vi "Non-Blocking Wait with Abort -- JKI SM Example.vi"() -> ()   [LabVIEW 2013]
panel:
  out "Current State":string
  out "Wait Timer Elapsed":bool
  out "Time Remaining":u32
  in  "Recipe Run Time (s)":dbl
  in  "Stop":bool
  in  "Start":bool
  in  "Exit":bool
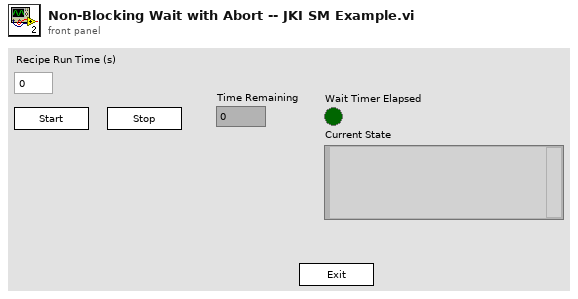
[diagram p1: front panel]
types:
  T1 = enum32{"Invalid", "Standard", "Closed", "Hidden", "Minimized", "Maximized"}
  T2 = enum32{"invalid app kind", "Development System", "Run Time System", "Student Edition", "Embedded LabVIEW", "Evaluation", "Custom"}
  T3 = cluster{"Core":cluster{"Current VI Reference":refnum<vi>, "Close Panel on Exit?":bool}, "Your Boolean data":bool, "Your string data":string}
  T4 = cluster{"Current VI Reference":refnum<vi>, "Close Panel on Exit?":bool}
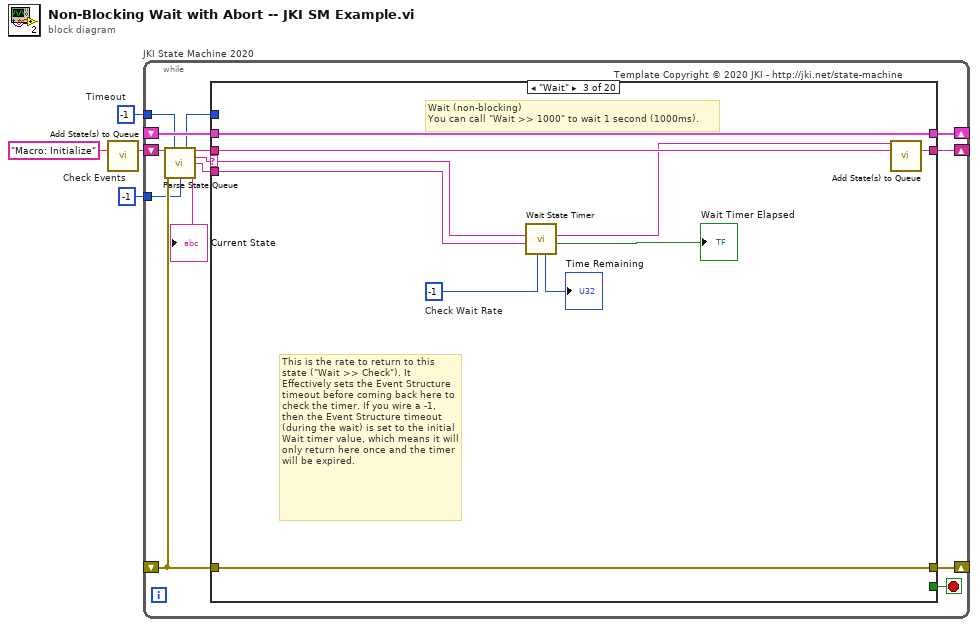
[diagram p0: block diagram]
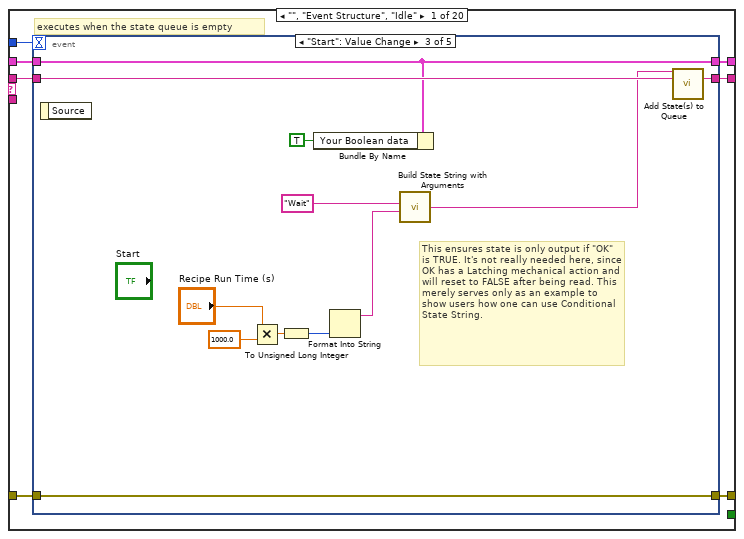
[diagram p2: hidden frame]
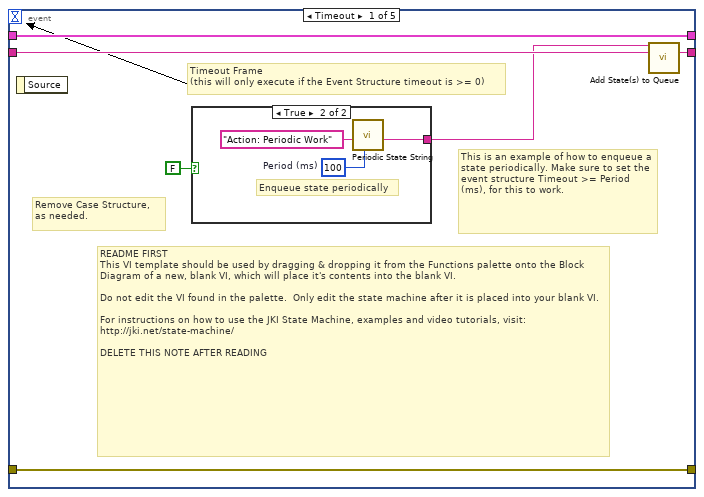
[diagram p3: hidden frame]
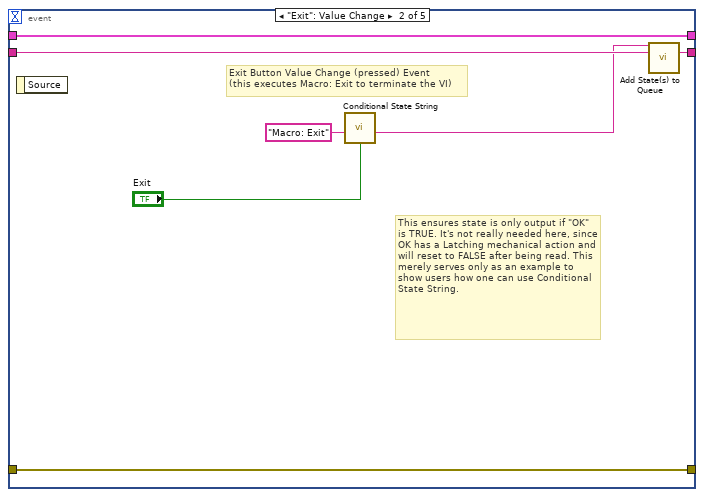
[diagram p5: hidden frame]
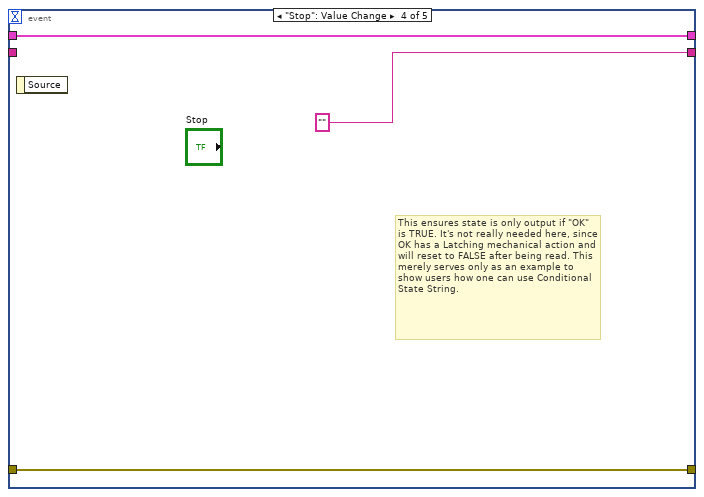
[diagram p6: hidden frame]
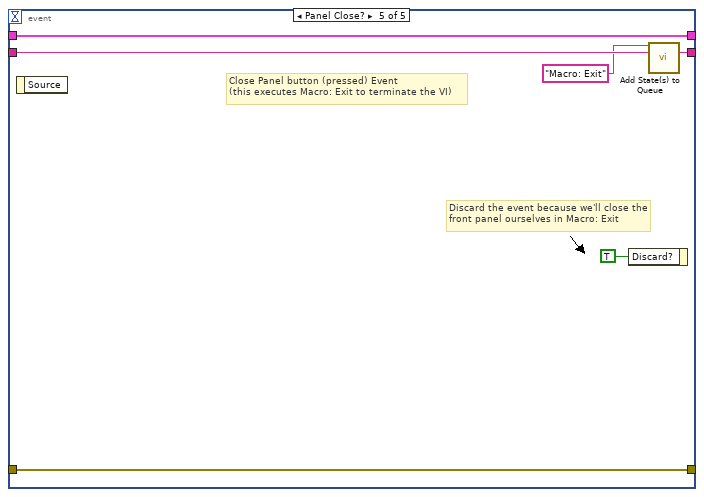
[diagram p7: hidden frame]
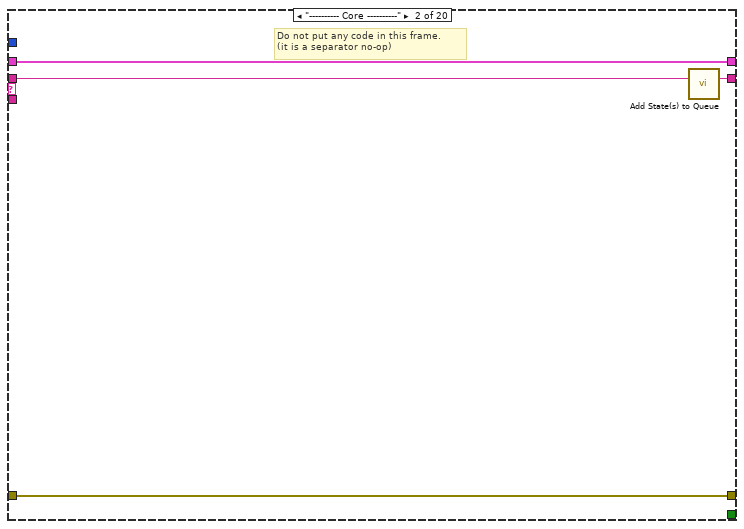
[diagram p8: hidden frame]
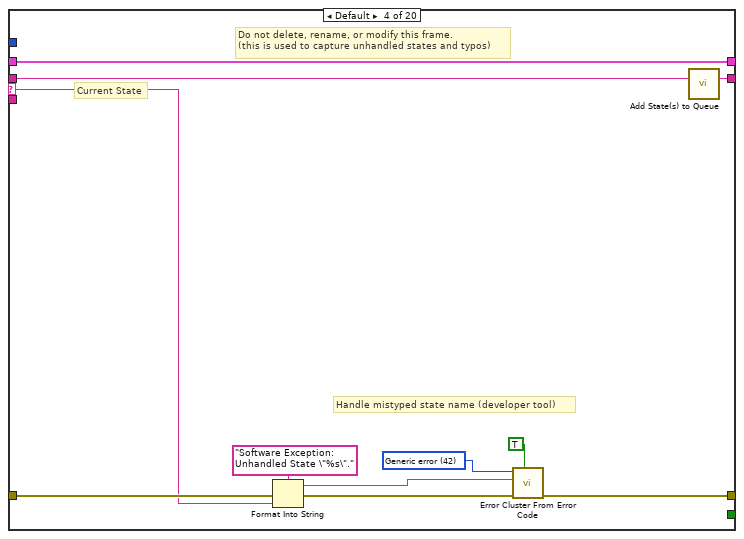
[diagram p9: hidden frame]
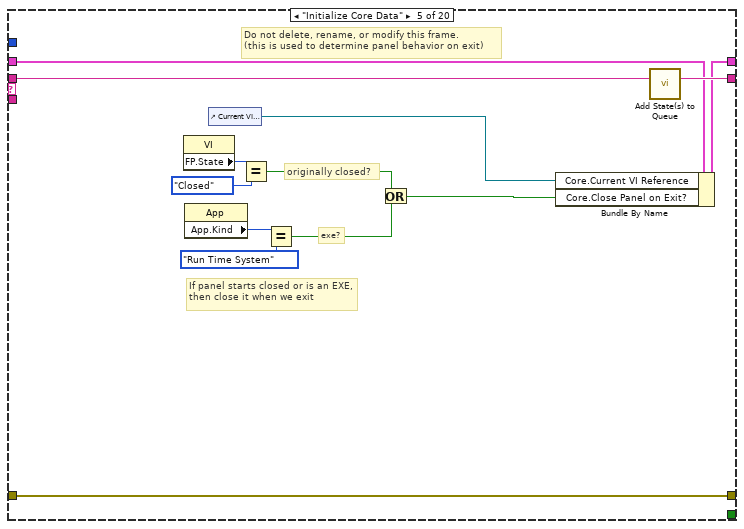
[diagram p10: hidden frame]
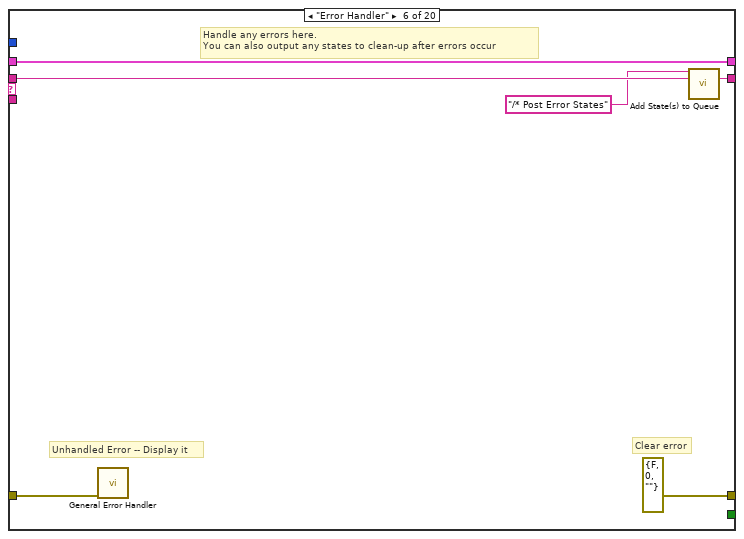
[diagram p11: hidden frame]
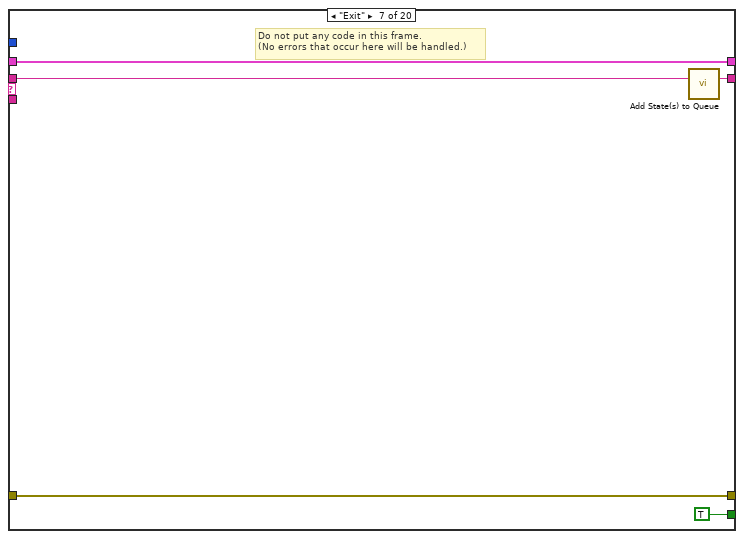
[diagram p12: hidden frame]
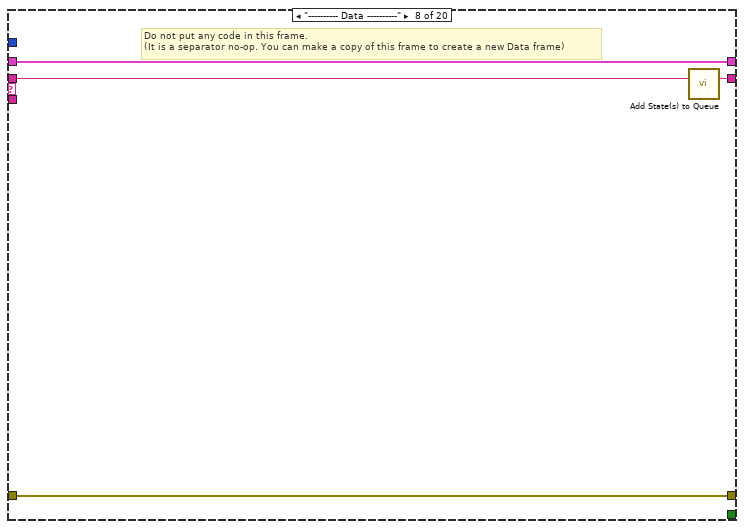
[diagram p13: hidden frame]
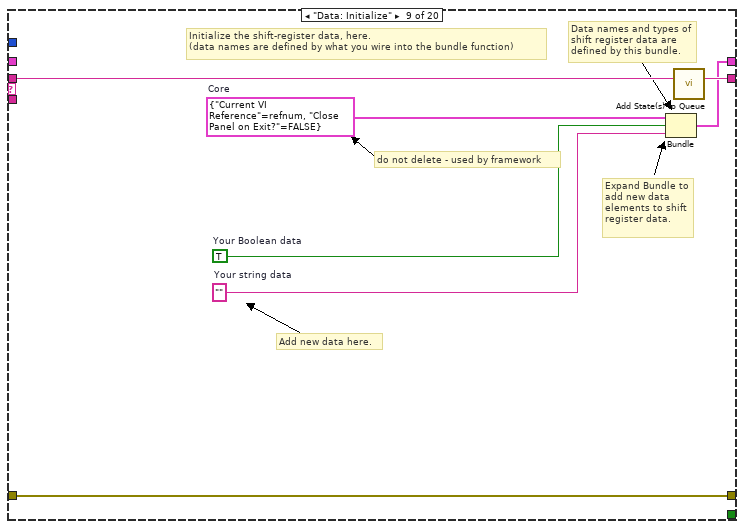
[diagram p14: hidden frame]
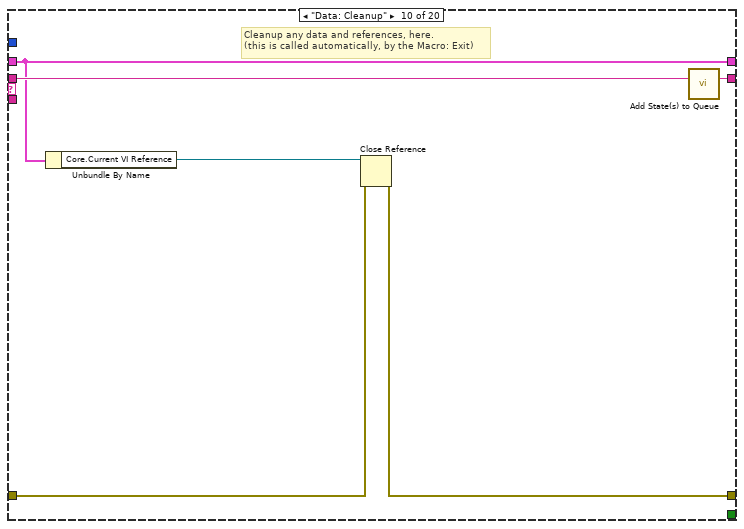
[diagram p15: hidden frame]
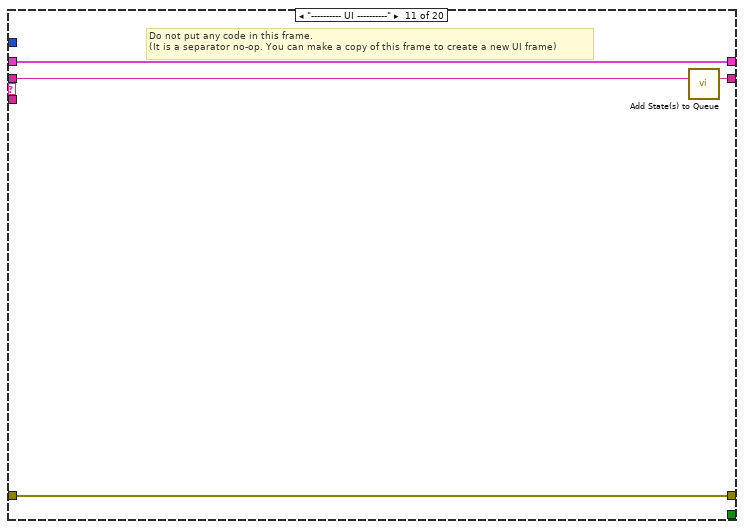
[diagram p16: hidden frame]
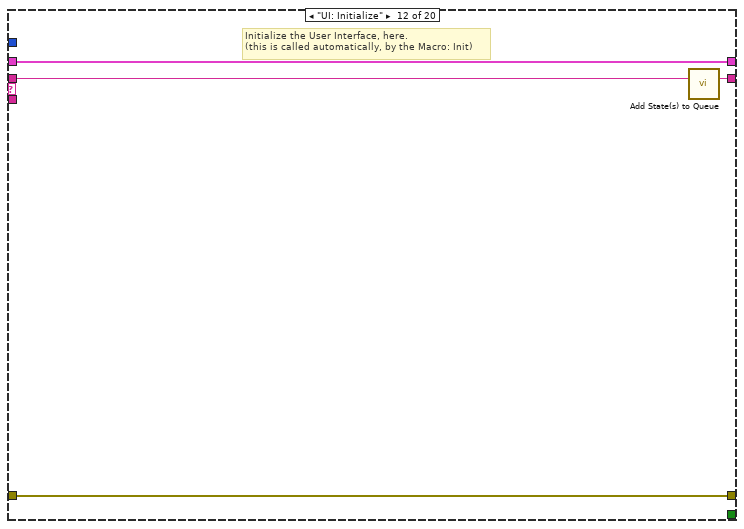
[diagram p17: hidden frame]
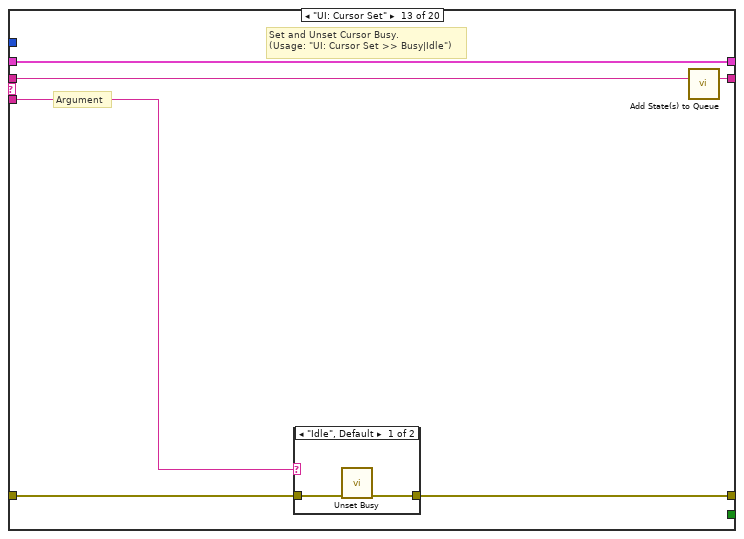
[diagram p18: hidden frame]
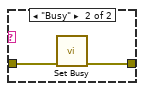
[diagram p19: hidden frame]
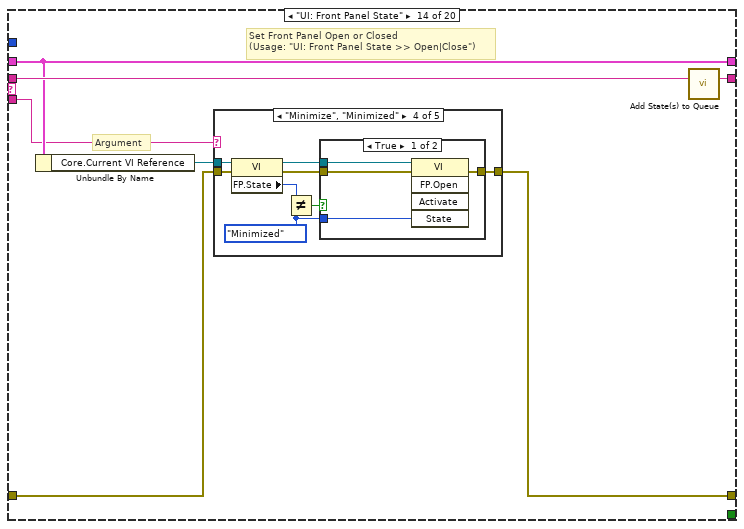
[diagram p20: hidden frame]
diagram:
  w1 = -1  # Check Events
  w2 = -1  # Timeout
  n1 = call "Add State(s) to Queue.vi"("State(s) in (\"\")"="Macro: Initialize") -> ("States Out"=w3:string)  [unwired: 14 in]
  n2 = while "JKI State Machine 2020" {
    shift-right: [w10] -> _
    shift-left: _ -> [w9]
    shift-right: [w13] -> _
    shift-left: _ -> [w8]
    shift-right: [w12] -> _
    shift-left: w3 -> [w14]
    tunnel: w2 -> [w7]
    tunnel: w1 -> [w5]
    stop <- w11 stop-if-true
    # "Template Copyright © 2020 JKI - http://jki.net/state-machine"
    n3 = call "Parse State Queue.vi"("State Queue"=w14, "Timeout"=w7, "Check Events rate"=w5, "Error In (no error)"=w8) -> ("Timeout out"=w6:i32, "Remaining States"=w16:string, "Current State"=w17:string, "Arguments"=w15:string)  [unwired: 8 in]
    "Current State" <- w17
    n4 = case shown="\"Wait\"" w17 {
      selector: w17 -> [_ _ w72 w76 _ _ _ _ _ _ _ _ _ _ _ _ _ _ _ _]
      tunnel: w16 -> [w24 w65 w75 w80 w99 w105 w110 w114 w121 w127 w131 w135 w141 w152 w221 w226 w236 w240 w244 w248]
      tunnel: w15 -> [_ _ w71 _ _ _ _ _ _ _ _ _ w136 w146 _ _ _ _ _ _]
      tunnel: w9 -> [w22 w62 w69 w78 w92 w102 w108 w111 _ w122 w128 w133 w139 w148 w218 w223 w233 w237 w241 w245]
      tunnel: [w21 w63 w73 w82 w96 errorcluster {"status"=FALSE, "code"=0, "source"=""} ("error out") w107 w112 w118 w123 w129 w132 w137 w149 w219 w224 w234 w238 w242 w246] -> w13
      tunnel: w8 -> [w20 w63 w73 w81 w96 w101 w107 w112 w118 w124 w129 w132 w138 w150 w219 w224 w234 w238 w242 w246]
      tunnel: [w23 w64 w74 w79 w98 w104 w109 w113 w120 w126 w130 w134 w140 w151 w220 w225 w235 w239 w243 w247] -> w12
      tunnel: [_ _ _ _ _ _ TRUE _ _ _ _ _ _ _ _ _ _ _ _ _] -> w11
      tunnel: [w19 w62 w69 w78 w97 w102 w108 w111 w119 w122 w128 w133 w139 w148 w218 w223 w233 w237 w241 w245] -> w10
      tunnel: w6 -> [w18 _ _ _ _ _ _ _ _ _ _ _ _ _ _ _ _ _ _ _]
      frame "", "Event Structure", "Idle" {
        # "executes when the state queue is empty"
        n5 = event shown="[2] \"Start\": Value Change" {
          selector: _ -> [_ _ _ _ _]
          dyn-events: _ -> [_ _ _ _ _]
          timeout: w18 -> [_ _ _ _ _]
          tunnel: w24 -> [w30 w40 w52 _ w61]
          tunnel: [w29 w39 w51 "" w60] -> w23
          tunnel: w22 -> [w27 w37 w42 w54 w58]
          tunnel: [w28 w38 w50 w55 w59] -> w21
          tunnel: w20 -> [w28 w38 w50 w55 w59]
          tunnel: [w27 w37 w42 w54 w58] -> w19
          event Timeout {
            # "Remove Case Structure, as needed."
            # "This is an example of how to enqueue a state periodically. Make sure to set the event structure Timeout >= Period (ms), for this to work."
            # "README FIRST\nThis VI template should be used by dragging & dropping it from the Functions palette onto the Block Diagram of a new, blank VI, which will place it's contents into the blank VI.\n\nDo not edit the VI found in the palette.  Only edit the state machine after it is placed into your blank VI.\n\nFor instructions on how to use the JKI State Machine, examples and video tutorials, visit:\nhttp://jki.net/state-machine/\n\nDELETE THIS NOTE AFTER READING"
            # "Timeout Frame\n(this will only execute if the Event Structure timeout is >= 0)"
            n6 = event-data() -> ()  [unwired: 1 in, 1 out]
            n7 = case shown="True" FALSE {
              tunnel: [_ w33] -> w26
              frame False {
              }
              frame True {
                w31 = u32 100  # Period (ms)
                # "Enqueue state periodically"
                n8 = call "Periodic State String.vi"("Period (ms)"=w31, "State"="Action: Periodic Work") -> ("State Out"=w33:string)  [unwired: 9 in]
              }
            }
            n9 = call "Add State(s) to Queue.vi"("State(s) in Front (\"\")"=w26, "State(s) in (\"\")"=w30) -> ("States Out"=w29:string)  [unwired: 13 in]
          }
          event "Exit": Value Change {
            # "This ensures state is only output if \"OK\" is TRUE. It's not really needed here, since OK has a Latching mechanical action and will reset to FALSE after being read. This merely serves only as an example to show users how one can use Conditional State String."
            # "Exit Button Value Change (pressed) Event\n(this executes Macro: Exit to terminate the VI)"
            n10 = event-data() -> ()  [unwired: 1 in, 1 out]
            n11 = call "Conditional State String.vi"("Do State(s)?"="Exit", "State"="Macro: Exit") -> ("State Out"=w34:string)  [unwired: 7 in]
            n12 = call "Add State(s) to Queue.vi"("State(s) in Front (\"\")"=w34, "State(s) in (\"\")"=w40) -> ("States Out"=w39:string)  [unwired: 13 in]
          }
          event "Start": Value Change {
            # "This ensures state is only output if \"OK\" is TRUE. It's not really needed here, since OK has a Latching mechanical action and will reset to FALSE after being read. This merely serves only as an example to show users how one can use Conditional State String."
            n13 = event-data() -> ()  [unwired: 1 in, 1 out]
            n14 = Multiply(x="Recipe Run Time (s)", y=1000.0) -> (x*y=w46:dbl)
            n15 = To Unsigned Long Integer(number=w46) -> (unsigned 32bit integer=w45:u32)
            n16 = Bundle By Name(cluster=w42, "Your Boolean data"=TRUE) -> ()  [unwired: 1 out]
            n17 = Format Into String(w45) -> (resulting string=w44:string)  [unwired: 3 in, 1 out]
            n18 = call "Build State String with Arguments.vi"("Arguments (\"\")"=w44, "State"="Wait") -> ("State with Arguments"=w43:string)  [unwired: 4 in]
            n19 = call "Add State(s) to Queue.vi"("State(s) in Front (\"\")"=w43, "State(s) in (\"\")"=w52) -> ("States Out"=w51:string)  [unwired: 13 in]
          }
          event "Stop": Value Change {
            # "This ensures state is only output if \"OK\" is TRUE. It's not really needed here, since OK has a Latching mechanical action and will reset to FALSE after being read. This merely serves only as an example to show users how one can use Conditional State String."
            n20 = event-data() -> ()  [unwired: 1 in, 1 out]
          }
          event Panel Close? {
            # "Discard the event because we'll close the front panel ourselves in Macro: Exit"
            # "Close Panel button (pressed) Event\n(this executes Macro: Exit to terminate the VI)"
            n21 = event-data() -> ()  [unwired: 1 in, 1 out]
            n22 = event-data("Discard?"=TRUE) -> ()  [unwired: 1 in, 1 out]
            n23 = call "Add State(s) to Queue.vi"("State(s) in Front (\"\")"="Macro: Exit", "State(s) in (\"\")"=w61) -> ("States Out"=w60:string)  [unwired: 13 in]
          }
        }
      }
      frame "---------- Core ----------" {
        # "Do not put any code in this frame.\n(it is a separator no-op)"
        n24 = call "Add State(s) to Queue.vi"("State(s) in (\"\")"=w65) -> ("States Out"=w64:string)  [unwired: 14 in]
      }
      frame "Wait" {
        w67 = -1  # Check Wait Rate
        # "This is the rate to return to this state (\"Wait >> Check\"). It Effectively sets the Event Structure timeout before coming back here to check the timer. If you wire a -1, then the Event Structure timeout (during the wait) is set to the initial Wait timer value, which means it will only return here once and the timer will be expired."
        # "Wait (non-blocking)\nYou can call \"Wait >> 1000\" to wait 1 second (1000ms)."
        n25 = call "Wait State Timer.vi"("Check Wait Rate"=w67, "Wait Time (Decimal String)"=w71, "Current State"=w72) -> ("Wait Timer Elapsed"=→"Wait Timer Elapsed":bool, "States to Enqueue"=w70:string, "Time Remaining"=→"Time Remaining":u32)  [unwired: 5 in, 1 out]
        n26 = call "Add State(s) to Queue.vi"("State(s) in Front (\"\")"=w70, "State(s) in (\"\")"=w75) -> ("States Out"=w74:string)  [unwired: 13 in]
      }
      frame Default {
        w85 = 42 items=["No error", "Argument error", "Memory is full", "Out of zone", "End of file", "File already open", "Generic file I/O error", "File not found", "File permission error", "Disk is full", "Duplicate path", "Too many files open", "System feature not enabled", "Resource file not found", "Cannot add resource", "Resource not found", "Image not found", "Image memory error", "Pen does not exist", "Config type invalid", "Config token not found", "Config parse error", "Config memory error", "Bad external code format", "Bad external code offset", "External code not present", "Null window", "Destroy window error", "Null menu", "Print aborted", "Bad print record", "Print driver error", "Windows error during printing", "Memory error during printing", "Print dialog error", "Generic print error", "Invalid device refnum", "Device not found", "Device parameter error", "Device unit error", "Cannot open device", "Device call aborted", "Generic error", "Cancelled by user", "Object ID too low", "Object ID too high", "Object not in heap", "Unknown heap", "Unknown object (invalid DefProc)", "Unknown object (DefProc not in table)", "Message out of range", "Invalid (null) method", "Unknown message", "Manager call not supported", "Bad address", "Network operation in progress", "Network operation timed out", "Connection is busy", "Network attribute not supported", "Network error", "Address in use", "System out of memory", "Connection aborted", "Connection refused", "Not connected", "Already connected", "Connection closed", "Initialization error (interapplication manager)", "Bad occurrence", "Wait on unbound occurrence handler", "Occurrence queue overflow", "Datalog type conflict", "Unused", "Unrecognized type (interapplication manager)", "Memory corrupt", "Failed to make temporary DLL", "Old CIN version", "Drag socket not found", "Failed to load drop-object", "Failed to register OLE object", "Failed to release OLE object", "Format specifier type mismatch", "Unknown format specifier", "Too few format specifiers", "Too many format specifiers", "Scan failed", "Newer CIN version", "Error converting to variant", "Runtime menu error", "Password tampered", "Variant attribute not found", "Incompatible variant data type", "Event data is not available", "Event Store is not present", "Occurrence is not found", "Event Queue is not created", "Event info is not available", "Refnum passed is NULL", "Error retrieving Class GUID", "Error retrieving CoClass GUID", "Error retrieving TypeLib GUID.", "Bad built application magic bytes.", "Specific driver is different from the specific driver associated with the Logical Name.", "There is no session opened to the class driver.", "Max Error", "MAX - Error with config objects", "MAX - Error loading configuration", "MAX - Group not supported"]
        # "Current State"
        # "Do not delete, rename, or modify this frame.\n(this is used to capture unhandled states and typos)"
        # "Handle mistyped state name (developer tool)"
        n27 = Format Into String(format string="Software Exception: Unhandled State \"%s\"." ("message"), error in=w81, w76) -> (resulting string=w84:string, error out=w83:errorcluster)  [unwired: 1 in]
        n28 = call <vilib>:"Error Cluster From Error Code.vi"("show call chain? (False)"=TRUE, "error in (no error)"=w83, "error message (\"\")"=w84, "error code (0)"=w85) -> ("error out"=w82:errorcluster)  [unwired: 5 in]
        n29 = call "Add State(s) to Queue.vi"("State(s) in (\"\")"=w80) -> ("States Out"=w79:string)  [unwired: 14 in]
      }
      frame "Initialize Core Data" {
        # "Do not delete, rename, or modify this frame.\n(this is used to determine panel behavior on exit)"
        # "originally closed?"
        # "exe?"
        # "If panel starts closed or is an EXE, then close it when we exit"
        n30 = property class="VI"() -> ("FP.State"=w89:T1)  [unwired: 2 in, 2 out]
        n31 = property class="App"() -> ("App.Kind"=w95:T2)  [unwired: 2 in, 2 out]
        n32 = control-ref of="Current VI Reference"() -> (w90:refnum<vi>)
        n33 = Equal?(x=w89, y=T1."Closed" ("Front Panel Window:State")) -> (x = y?=w87:bool)
        n34 = Equal?(x=w95, y=T2."Run Time System" ("Application:Kind")) -> (x = y?=w93:bool)
        n35 = Or(x=w87, y=w93) -> (x .or. y?=w91:bool)
        n36 = Bundle By Name(cluster=w92, "Core.Current VI Reference"=w90, "Core.Close Panel on Exit?"=w91) -> (w97:T3)
        n37 = call "Add State(s) to Queue.vi"("State(s) in (\"\")"=w99) -> ("States Out"=w98:string)  [unwired: 14 in]
      }
      frame "Error Handler" {
        # "Unhandled Error -- Display it"
        # "Handle any errors here.\nYou can also output any states to clean-up after errors occur"
        # "Clear error"
        n38 = call <vilib>:"General Error Handler.vi"("error in (no error)"=w101) -> ()  [unwired: 10 in, 5 out]
        n39 = call "Add State(s) to Queue.vi"("State(s) in Front (\"\")"="/* Post Error States", "State(s) in (\"\")"=w105) -> ("States Out"=w104:string)  [unwired: 13 in]
      }
      frame "Exit" {
        # "Do not put any code in this frame.\n(No errors that occur here will be handled.)"
        n40 = call "Add State(s) to Queue.vi"("State(s) in (\"\")"=w110) -> ("States Out"=w109:string)  [unwired: 14 in]
      }
      frame "---------- Data ----------" {
        # "Do not put any code in this frame.\n(It is a separator no-op. You can make a copy of this frame to create a new Data frame)"
        n41 = call "Add State(s) to Queue.vi"("State(s) in (\"\")"=w114) -> ("States Out"=w113:string)  [unwired: 14 in]
      }
      frame "Data: Initialize" {
        w115 = T4 {"Current VI Reference"=refnum, "Close Panel on Exit?"=FALSE}  # Core
        w117 = TRUE  # Your Boolean data
        w116 = ""  # Your string data
        # "do not delete - used by framework"
        # "Expand Bundle to add new data elements to shift register data."
        # "Add new data here."
        # "Data names and types of shift register data are defined by this bundle."
        # "Initialize the shift-register data, here.\n(data names are defined by what you wire into the bundle function)"
        n42 = Bundle("Core"=w115, "Your Boolean data"=w117, "Your string data"=w116) -> (w119:T3)  [unwired: 1 in]
        n43 = call "Add State(s) to Queue.vi"("State(s) in (\"\")"=w121) -> ("States Out"=w120:string)  [unwired: 14 in]
      }
      frame "Data: Cleanup" {
        # "Cleanup any data and references, here.\n(this is called automatically, by the Macro: Exit)"
        n44 = Unbundle By Name(w122) -> ("Core.Current VI Reference"=w125:refnum<vi>)
        n45 = Close Reference(reference=w125, error in (no error)=w124) -> (error out=w123:errorcluster)
        n46 = call "Add State(s) to Queue.vi"("State(s) in (\"\")"=w127) -> ("States Out"=w126:string)  [unwired: 14 in]
      }
      frame "---------- UI ----------" {
        # "Do not put any code in this frame.\n(It is a separator no-op. You can make a copy of this frame to create a new UI frame)"
        n47 = call "Add State(s) to Queue.vi"("State(s) in (\"\")"=w131) -> ("States Out"=w130:string)  [unwired: 14 in]
      }
      frame "UI: Initialize" {
        # "Initialize the User Interface, here.\n(this is called automatically, by the Macro: Init)"
        n48 = call "Add State(s) to Queue.vi"("State(s) in (\"\")"=w135) -> ("States Out"=w134:string)  [unwired: 14 in]
      }
      frame "UI: Cursor Set" {
        # "Argument"
        # "Set and Unset Cursor Busy.\n(Usage: \"UI: Cursor Set >> Busy|Idle\")"
        n49 = case shown="\"Idle\", Default" w136 {
          tunnel: w138 -> [w143 w145]
          tunnel: [w142 w144] -> w137
          frame "Idle", Default {
            n50 = call <vilib>:"Unset Busy.vi"("error in (no error)"=w143) -> ("error out"=w142:errorcluster)  [unwired: 10 in]
          }
          frame "Busy" {
            n51 = call <vilib>:"Set Busy.vi"("error in (no error)"=w145) -> ("error out"=w144:errorcluster)  [unwired: 9 in, 1 out]
          }
        }
        n52 = call "Add State(s) to Queue.vi"("State(s) in (\"\")"=w141) -> ("States Out"=w140:string)  [unwired: 14 in]
      }
      frame "UI: Front Panel State" {
        # "Argument"
        # "Set Front Panel Open or Closed\n(Usage: \"UI: Front Panel State >> Open|Close\")"
        n53 = Unbundle By Name(w148) -> ("Core.Current VI Reference"=w147:refnum<vi>)
        n54 = case shown="\"Minimize\", \"Minimized\"" w146 {
          tunnel: w150 -> [w158 w173 w184 w197 w210]
          tunnel: [w160 w174 w186 w199 w212] -> w149
          tunnel: w147 -> [w159 w171 w185 w198 w211]
          frame "Open", "Standard", Default {
            w153 = T1."Standard" ("State")
            n55 = property class="VI"(reference=w159, error in=w158) -> (reference out=w156:refnum<vi>, error out=w157:errorcluster, "FP.State"=w155:T1)
            n56 = Not Equal?(x=w155, y=w153) -> (x != y?=w154:bool)
            n57 = case shown="True" w154 {
              tunnel: [w164 w166] -> w160
              tunnel: w157 -> [w163 w166]
              tunnel: w156 -> [w162 _]
              tunnel: w153 -> [w161 _]
              frame True {
                n58 = invoke class="VI" method="FP.Open"(reference=w162, error in=w163, "Activate"=TRUE, "State"=w161) -> (error out=w164:errorcluster)  [unwired: 1 in, 4 out]
              }
              frame False {
              }
            }
          }
          frame "Close", "Closed" {
            n59 = property class="VI"(reference=w171, error in=w173) -> (reference out=w170:refnum<vi>, error out=w172:errorcluster, "FP.State"=w168:T1)
            n60 = Not Equal?(x=w168, y=T1."Closed" ("Front Panel Window:State")) -> (x != y?=w167:bool)
            n61 = case shown="True" w167 {
              tunnel: [w175 w178] -> w174
              tunnel: w172 -> [w175 w177]
              tunnel: w170 -> [_ w176]
              frame False {
              }
              frame True {
                n62 = invoke class="VI" method="FP.Close"(reference=w176, error in=w177) -> (error out=w178:errorcluster)  [unwired: 1 in, 2 out]
              }
            }
          }
          frame "Hidden", "Hide" {
            w179 = T1."Hidden" ("State")
            n63 = property class="VI"(reference=w185, error in=w184) -> (reference out=w182:refnum<vi>, error out=w183:errorcluster, "FP.State"=w181:T1)
            n64 = Not Equal?(x=w181, y=w179) -> (x != y?=w180:bool)
            n65 = case shown="True" w180 {
              tunnel: [w190 w191] -> w186
              tunnel: w183 -> [w189 w191]
              tunnel: w182 -> [w188 _]
              tunnel: w179 -> [w187 _]
              frame True {
                n66 = invoke class="VI" method="FP.Open"(reference=w188, error in=w189, "State"=w187) -> (error out=w190:errorcluster)  [unwired: 2 in, 4 out]
              }
              frame False {
              }
            }
          }
          frame "Minimize", "Minimized" {
            w192 = T1."Minimized" ("State")
            n67 = property class="VI"(reference=w198, error in=w197) -> (reference out=w195:refnum<vi>, error out=w196:errorcluster, "FP.State"=w194:T1)
            n68 = Not Equal?(x=w194, y=w192) -> (x != y?=w193:bool)
            n69 = case shown="True" w193 {
              tunnel: [w203 w204] -> w199
              tunnel: w196 -> [w202 w204]
              tunnel: w195 -> [w201 _]
              tunnel: w192 -> [w200 _]
              frame True {
                n70 = invoke class="VI" method="FP.Open"(reference=w201, error in=w202, "State"=w200) -> (error out=w203:errorcluster)  [unwired: 2 in, 4 out]
              }
              frame False {
              }
            }
          }
          frame "Maximize", "Maximized" {
            w205 = T1."Maximized" ("State")
            n71 = property class="VI"(reference=w211, error in=w210) -> (reference out=w208:refnum<vi>, error out=w209:errorcluster, "FP.State"=w207:T1)
            n72 = Not Equal?(x=w207, y=w205) -> (x != y?=w206:bool)
            n73 = case shown="True" w206 {
              tunnel: [w216 w217] -> w212
              tunnel: w209 -> [w215 w217]
              tunnel: w208 -> [w214 _]
              tunnel: w205 -> [w213 _]
              frame True {
                n74 = invoke class="VI" method="FP.Open"(reference=w214, error in=w215, "State"=w213) -> (error out=w216:errorcluster)  [unwired: 2 in, 4 out]
              }
              frame False {
              }
            }
          }
        }
        n75 = call "Add State(s) to Queue.vi"("State(s) in (\"\")"=w152) -> ("States Out"=w151:string)  [unwired: 14 in]
      }
      frame "---------- Macro ----------" {
        # "Do not put any code in this frame.\n(It is a separator no-op. You can make a copy of this frame to create a new Macro frame)"
        n76 = call "Add State(s) to Queue.vi"("State(s) in (\"\")"=w221) -> ("States Out"=w220:string)  [unwired: 14 in]
      }
      frame "Macro: Initialize" {
        w222 = "Data: Initialize\nInitialize Core Data\nUI: Initialize\nUI: Front Panel State >> Open"  # Data: Initialize Initialize Core Data UI: Initialize UI: Front Panel State >> Open
        # "Initialization Macro\n(This is called once, when the VI starts)"
        n77 = call "Add State(s) to Queue.vi"("State(s) in Front (\"\")"=w222, "State(s) in (\"\")"=w226) -> ("States Out"=w225:string)  [unwired: 13 in]
      }
      frame "Macro: Exit" {
        # "Exit Macro\n(This is called once, when the VI exits)"
        n78 = Unbundle By Name(w233) -> ("Core.Close Panel on Exit?"=w232:bool)
        n79 = Select(t="UI: Front Panel State >> Close", s=w232, f="") -> (s? t:f=w229:string)
        n80 = call "Add State(s) to Queue.vi"("State(s) in (\"\")"=w229, "State(s) at Back (\"\")"="Data: Cleanup\nExit") -> ("States Out"=w227:string)  [unwired: 13 in]
        n81 = call "Add State(s) to Queue.vi"("State(s) in Front (\"\")"=w227, "State(s) in (\"\")"=w236) -> ("States Out"=w235:string)  [unwired: 13 in]
      }
      frame "---------- New Category ----------" {
        # "Template Separator\n(You can make a copy of, or modify, this frame)"
        n82 = call "Add State(s) to Queue.vi"("State(s) in (\"\")"=w240) -> ("States Out"=w239:string)  [unwired: 14 in]
      }
      frame "New Category: 1" {
        # "Your code here.\n(You can make a copy of, or modify, this frame)"
        n83 = call "Add State(s) to Queue.vi"("State(s) in (\"\")"=w244) -> ("States Out"=w243:string)  [unwired: 14 in]
      }
      frame "New Category: 2" {
        # "Your code here.\n(You can make a copy of, or modify, this frame)"
        n84 = call "Add State(s) to Queue.vi"("State(s) in (\"\")"=w248) -> ("States Out"=w247:string)  [unwired: 14 in]
      }
    }
  }
